vi "Select Page.vi"(8 "error in (no error)":errorcluster, 10 "Page":u32, 11 "BigMAQ in":refnum<class "BigMAQ.lvclass">) -> (0 "error out":errorcluster, 2 "Corrected Page":u32, 3 "BigMAQ out":refnum<class "BigMAQ.lvclass">)   [LabVIEW 2019, in "BigMAQ.lvclass"]
uses:
  BigMAQ.lvclass
  BigMAQ.lvclass/BigMAQ.ctl
  <vilib>/LabVIEW Open Source Project/Unicity/RandomStringGenerator/RandomStringGenerator.lvclass
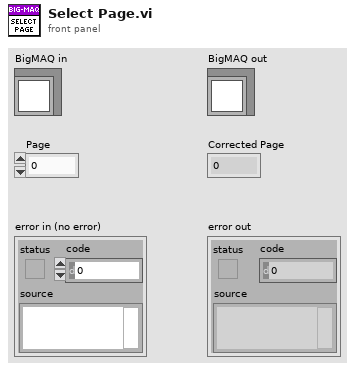
[diagram p1: front panel]
types:
  T1 = typedef "Image Type" = u32
  T2 = typedef "IMAQ Image.ctl" = refnum<image>
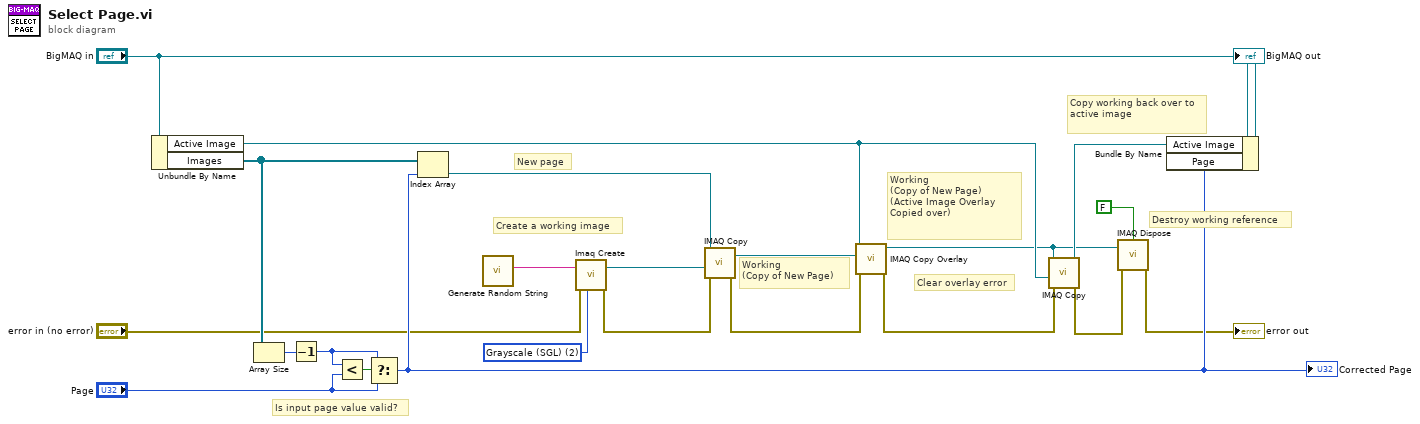
[diagram p0: block diagram]
diagram:
  w15 = T1 2 items=["Grayscale (U8)", "Grayscale (I16)", "Grayscale (SGL)", "Complex (CSG)", "RGB (U32)", "HSL (U32)", "RGB (U64)", "Grayscale (U16)"] ("Image Type")
  # "Clear overlay error"
  # "Is input page value valid?"
  # "New page"
  # "Create a working image"
  # "Destroy working reference"
  # "Copy working back over to active image"
  # "Working\n(Copy of New Page)\n(Active Image Overlay Copied over)"
  # "Working\n(Copy of New Page)"
  n1 = Unbundle By Name("BigMAQ in") -> ("Active Image"=w8:T2, "Images"=w18:T2[])
  n2 = Array Size(array=w18) -> (size(s)=w22:i32)
  n3 = Decrement(x=w22) -> (x-1=w20:i32)
  n4 = Less?(x=w20, y="Page") -> (x < y?=w21:bool)
  n5 = Select(t=w20, s=w21, f="Page") -> (s? t:f=w17:u32)
  "Corrected Page" <- w17
  n6 = Index Array(array=w18, index=w17) -> (element=w16:T2)
  n7 = call <vilib>:"Generate Random String.vi"() -> ("Random String"=w1:string)  [unwired: 11 in]
  n8 = call "Imaq Create"("Image Name"=w1, "Image Type"=w15, "error in (no error)"="error in (no error)") -> ("New Image"=w10:T2, "error out"=w12:errorcluster)  [unwired: 2 in]
  n9 = call "IMAQ Copy"("error in (no error)"=w12, "Image Dst"=w10, "Image Src"=w16) -> ("error out"=w11:errorcluster, "Image Dst Out"=w9:T2)  [unwired: 3 in]
  n10 = call "IMAQ Copy Overlay"("error in (no error)"=w11, "Image Dst"=w9, "Image Src"=w8) -> ("error out"=w3:errorcluster, "Image Dst Out"=w5:T2)  [unwired: 7 in]
  n11 = call "IMAQ Copy"("error in (no error)"=w3, "Image Dst"=w8, "Image Src"=w5) -> ("error out"=w13:errorcluster, "Image Dst Out"=w7:T2)  [unwired: 3 in]
  n12 = call "IMAQ Dispose"("All Images? (No)"=FALSE, "Image"=w5, "error in (no error)"=w13) -> ("error out"=→"error out":errorcluster)  [unwired: 3 in]
  n13 = Bundle By Name(cluster="BigMAQ in", "Active Image"=w7, "Page"=w17) -> (→"BigMAQ out":refnum<class "BigMAQ.lvclass">)
